vi "Dequeue.vi"(6 "abort (F)":bool, 8 "element in":T1, 11 "PipeData in":refnum<class "StreamData.lvclass">) -> (0 "element out":T1, 1 "count":i32, 2 "wait":refnum<k4>, 3 "PipeData out":refnum<class "StreamData.lvclass">, 4 "aborted?":bool, 5 "last element?":bool)   [LabVIEW 2017, in "Stream-t'WPI_EncoderType.ctl'.lvlib" / "StreamData.lvclass"]
uses:
  <extravilib>/ChannelInstances/Stream-t'WPI_EncoderType.ctl'/StreamData.lvclass
  <vilib>/Rock Robotics/WPI/Encoder/WPI_EncoderType.ctl
  <extravilib>/ChannelInstances/Stream-t'WPI_EncoderType.ctl'/StreamData.lvclass/StreamData.ctl
  <resource>/ChannelSupport/_ChannelSupport/PipeLogic/PipeLogic.lvclass/PipeLogic.ctl
  <resource>/ChannelSupport/_ChannelSupport/PipeLogic/PipeLogic.lvclass
  <resource>/ChannelSupport/_ChannelSupport/_ChannelSupport.lvlib
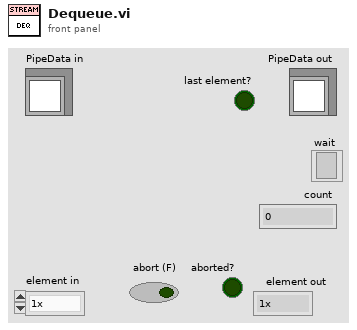
[diagram p1: front panel]
types:
  T1 = typedef "WPI_EncoderType.ctl" = enum16{"1x", "2x", "4x"}
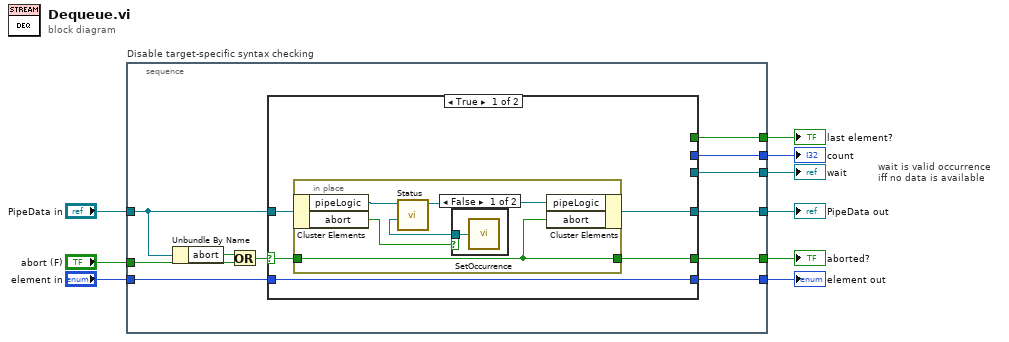
[diagram p0: block diagram]
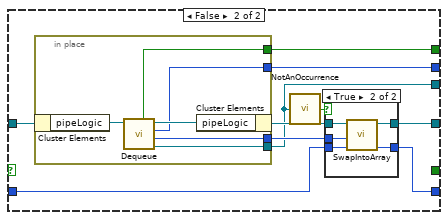
[diagram p3: hidden frame]
diagram:
  # "wait is valid occurrence\niff no data is available"
  n1 = stacked-sequence "Disable target-specific syntax checking" {
    tunnel: [w20] -> w9
    tunnel: [w19] -> w8
    tunnel: [w18] -> w7
    tunnel: [w17] -> w6
    tunnel: [w16] -> w5
    tunnel: [w15] -> w4
    tunnel: "element in" -> [w14]
    tunnel: "PipeData in" -> [w13]
    tunnel: "abort (F)" -> [w11]
    frame #0 {
      n2 = Unbundle By Name(w13) -> ("abort"=w12:bool)
      n3 = Or(x=w12, y=w11) -> (x .or. y?=w10:bool)
      n4 = case shown="True" w10 {
        selector: w10 -> [w22 _]
        tunnel: w13 -> [w25 w41]
        tunnel: [w24 w38] -> w20
        tunnel: [_ w40] -> w19
        tunnel: [_ w39] -> w18
        tunnel: [w23 _] -> w17
        tunnel: [w21 w36] -> w16
        tunnel: [_ w33] -> w15
        tunnel: w14 -> [w21 w35]
        frame True {
          n5 = in-place {
            in-place-border: [w27] -> w23
            in-place-border: w22 -> [w27]
            n6 = in-place-cluster #1(w25) -> ("pipeLogic"=w30:refnum<class "PipeLogic.lvclass">, "abort"=w28:bool)
            n7 = call <resource>:"Status.vi"("pipeLogic in"=w30) -> ("pipeLogic out"=w29:refnum<class "PipeLogic.lvclass">, "nonFull"=w26:refnum<k4>)  [unwired: 2 in, 7 out]
            n8 = case shown="False" w28 {
              tunnel: w26 -> [w31 _]
              frame False {
                n9 = call <resource>:"SetOccurrence.vi"("occurrence"=w31) -> ()  [unwired: 9 in]
              }
              frame True {
              }
            }
            n10 = in-place-cluster #1("pipeLogic"=w29, "abort"=w27) -> (w24:refnum<class "StreamData.lvclass">)
          }
        }
        frame False {
          n11 = in-place {
            in-place-border: [w49] -> w33
            in-place-border: [w52] -> w39
            in-place-border: [w51] -> w40
            in-place-border: [w50] -> w34
            n12 = in-place-cluster #2(w41) -> ("pipeLogic"=w54:refnum<class "PipeLogic.lvclass">)
            n13 = call <resource>:"Dequeue.vi"("pipeLogic in"=w54) -> ("wait"=w49:refnum<k4>, "index"=w50:i32, "count"=w52:i32, "pipeLogic out"=w53:refnum<class "PipeLogic.lvclass">, "last element out"=w51:bool)  [unwired: 6 in]
            n14 = in-place-cluster #2("pipeLogic"=w53) -> (w37:refnum<class "StreamData.lvclass">)
          }
          n15 = call <resource>:"NotAnOccurrence.vi"("occurrence refnum"=w33) -> ("not an occurrence?"=w32:bool)
          n16 = case shown="True" w32 {
            tunnel: [w43 w47] -> w38
            tunnel: w37 -> [w43 w48]
            tunnel: w35 -> [w42 w46]
            tunnel: [w42 w45] -> w36
            tunnel: w34 -> [_ w44]
            frame False {
            }
            frame True {
              n17 = call <extravilib>:"SwapIntoArray.vi"("element in"=w46, "index"=w44, "PipeData in"=w48) -> ("element out"=w45:T1, "PipeData out"=w47:refnum<class "StreamData.lvclass">)  [unwired: 7 in]
            }
          }
        }
      }
    }
  }
  "PipeData out" <- w9
  "aborted?" <- w6
  "last element?" <- w8
  "count" <- w7
  "wait" <- w4
  "element out" <- w5
